vi "ryTimerEx UserEvent.vi"() -> ()   [LabVIEW 2020]
uses:
  1f272512-79a9-4561-a15c-77982c9f9615.vi
  Lib/ryTimer.lvclass
panel:
  in  "Wait Time ms (0=Use existing)":u32
  in  "Start":bool
  in  "Stop":bool
  out "dT (ms)":u32
  out "Counter":u32
  out "Event":string
  out "Last Sent (ms)":u32
  out "Wait Time (ms)":u32
  out "Is Running?":bool
  out "Time Left (ms)":i32
  in  "Exit":bool
  out "Error":errorcluster
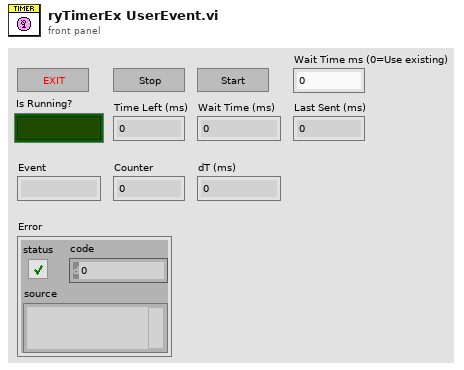
[diagram p1: front panel]
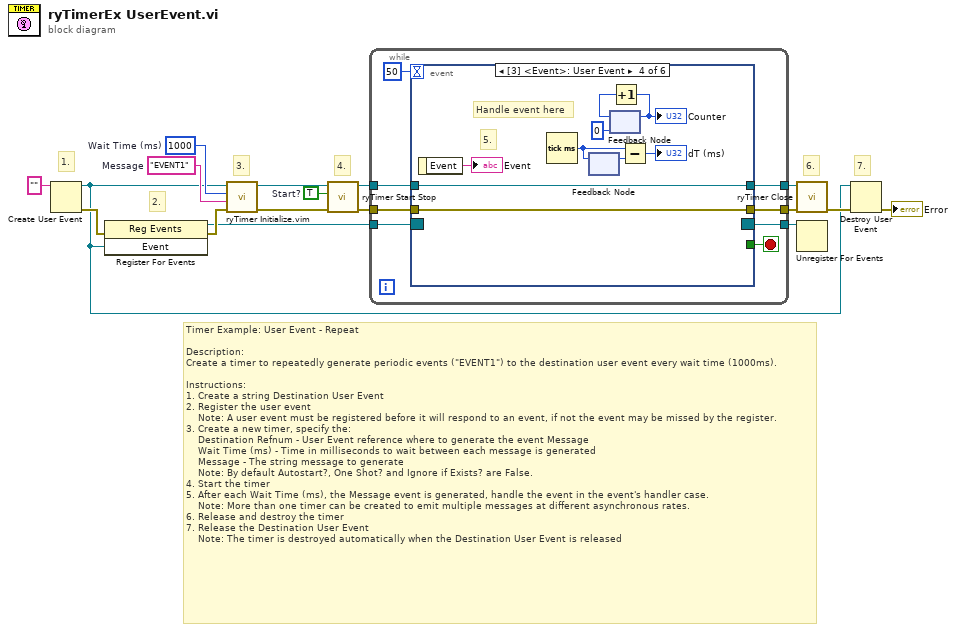
[diagram p0: block diagram]
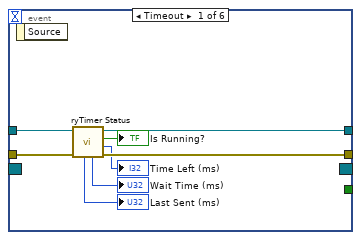
[diagram p2: hidden frame]
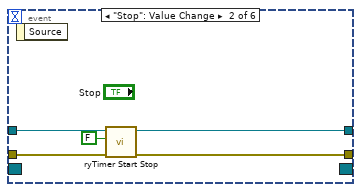
[diagram p3: hidden frame]
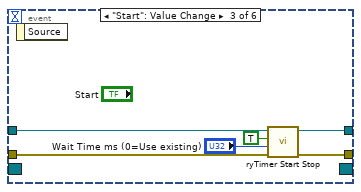
[diagram p4: hidden frame]
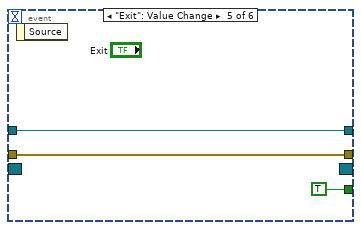
[diagram p5: hidden frame]
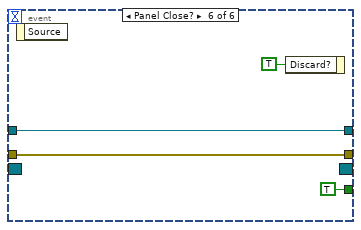
[diagram p6: hidden frame]
diagram:
  w3 = TRUE  # Start?
  w15 = "EVENT1"  # Message
  w16 = u32 1000  # Wait Time (ms)
  # "Timer Example: User Event - Repeat\n\nDescription:\nCreate a timer to repeatedly generate periodic events (\"EVENT1\") to the destination user event every wait time (1000ms).\n\nInstructions:\n1. Create a string Destination User Event\n2. Register the user event\n    Note: A user event must be registered before it will respond to an event, if not the event may be missed by the register.\n3. Create a new timer, specify the:\n    Destination Refnum - User Event reference where to generate the event Message\n    Wait Time (ms) - Time in milliseconds to wait between each message is generated\n    Message - The string message to generate\n    Note: By default Autostart?, One Shot? and Ignore if Exists? are False.\n4. Start the timer\n5. After each Wait Time (ms), the Message event is generated, handle the event in the event's handler case.\n    Note: More than one timer can be created to emit multiple messages at different asynchronous rates.\n6. Release and destroy the timer\n7. Release the Destination User Event\n    Note: The timer is destroyed automatically when the Destination User Event is released"
  # "7."
  # "6."
  # "4."
  # "3."
  # "2."
  # "1."
  n1 = Create User Event(user event datatype="" ("Event")) -> (user event=w1:refnum<user-event>, error out=w14:errorcluster)  [unwired: 1 in]
  n2 = register-events(error in=w14, w1) -> (reference out=w12:refnum<event-registration>, error out=w13:errorcluster)  [unwired: 1 in]
  n3 = call "ryTimer Initialize.vim"("error in (no error)"=w13, "Message"=w15, "Wait Time (ms)"=w16, "Destination Refnum [Q,UE,Any]"=w1) -> ("error out"=w7:errorcluster, "Timer out"=w5:refnum<class "ryTimer.lvclass">)  [unwired: 6 in]
  n4 = call "ryTimer Start Stop.vi"("error in (no error)"=w7, "Start? (F=Stop)"=w3, "Timer in"=w5) -> ("error out"=w6:errorcluster, "Timer out"=w4:refnum<class "ryTimer.lvclass">)  [unwired: 7 in]
  n5 = while {
    tunnel: w6 -> [w25]
    tunnel: w12 -> [w24]
    tunnel: w4 -> [w23]
    tunnel: [w21] -> w10
    tunnel: [w20] -> w11
    tunnel: [w19] -> w9
    stop <- w18 stop-if-true
    n6 = event shown="[3] <Event>: User Event" {
      selector: w24 -> [_ _ _ _ _ _]
      dyn-events: [_ _ _ _ _ _] -> w19
      timeout: 50 -> [_ _ _ _ _ _]
      tunnel: w25 -> [w32 w37 w43 w52 w55 w58]
      tunnel: w23 -> [w30 w38 w44 w53 w56 w60]
      tunnel: [w33 w36 w42 w52 w55 w58] -> w21
      tunnel: [w31 w35 w41 w53 w56 w60] -> w20
      tunnel: [_ _ _ _ TRUE TRUE] -> w18
      event Timeout {
        n7 = event-data() -> ()  [unwired: 1 in, 1 out]
        n8 = call "ryTimer Status.vi"("error in (no error)"=w32, "Timer in"=w30) -> ("error out"=w33:errorcluster, "Time Left (ms) [-1=Unknown]"=→"Time Left (ms)":i32, "Is Running?"=→"Is Running?":bool, "Timer out"=w31:refnum<class "ryTimer.lvclass">, "Wait Time (ms)"=→"Wait Time (ms)":u32, "Last Ticks (ms)"=→"Last Sent (ms)":u32)  [unwired: 4 in]
      }
      event "Stop": Value Change {
        n9 = event-data() -> ()  [unwired: 1 in, 1 out]
        n10 = call "ryTimer Start Stop.vi"("error in (no error)"=w37, "Start? (F=Stop)"=FALSE, "Timer in"=w38) -> ("error out"=w36:errorcluster, "Timer out"=w35:refnum<class "ryTimer.lvclass">)  [unwired: 7 in]
      }
      event "Start": Value Change {
        n11 = event-data() -> ()  [unwired: 1 in, 1 out]
        n12 = call "ryTimer Start Stop.vi"("error in (no error)"=w43, "Wait Time ms (0=Use existing)"="Wait Time ms (0=Use existing)", "Start? (F=Stop)"=TRUE, "Timer in"=w44) -> ("error out"=w42:errorcluster, "Timer out"=w41:refnum<class "ryTimer.lvclass">)  [unwired: 6 in]
      }
      event User Event {
        # "5."
        # "Handle event here"
        n13 = event-data() -> ("Event"=→"Event":string)  [unwired: 1 in]
        n14 = Tick Count (ms)() -> (millisecond timer value=w47:u32)
        n15 = feedback #1() -> (w46:u32)  [unwired: 1 in]
        n16 = feedback-in #1(w47) -> ()
        n17 = feedback #2(u32 0) -> (w49:u32)
        n18 = Increment(x=w49) -> (x+1=w48:u32)
        "Counter" <- w48
        n19 = feedback-in #2(w48) -> ()
        n20 = Subtract(x=w47, y=w46) -> (x-y=→"dT (ms)":u32)
      }
      event "Exit": Value Change {
        n21 = event-data() -> ()  [unwired: 1 in, 1 out]
      }
      event Panel Close? {
        n22 = event-data() -> ()  [unwired: 1 in, 1 out]
        n23 = event-data("Discard?"=TRUE) -> ()  [unwired: 1 in, 1 out]
      }
    }
  }
  n24 = call "ryTimer Close.vi"("error in (no error)"=w10, "Timer in"=w11) -> ("error out"=w8:errorcluster)  [unwired: 9 in]
  n25 = Unregister For Events(event registration refnum=w9) -> ()  [unwired: 1 in, 1 out]
  n26 = Destroy User Event(user event=w1, error in=w8) -> (error out=→"Error":errorcluster)
